vi "HGB2-SpeedControl_Rev00.vi"(11 "Set Speed":dbl format="%#_13g") -> (3 "Speed Control Output":dbl)   [LabVIEW 2016]
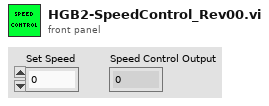
[diagram p1: front panel]
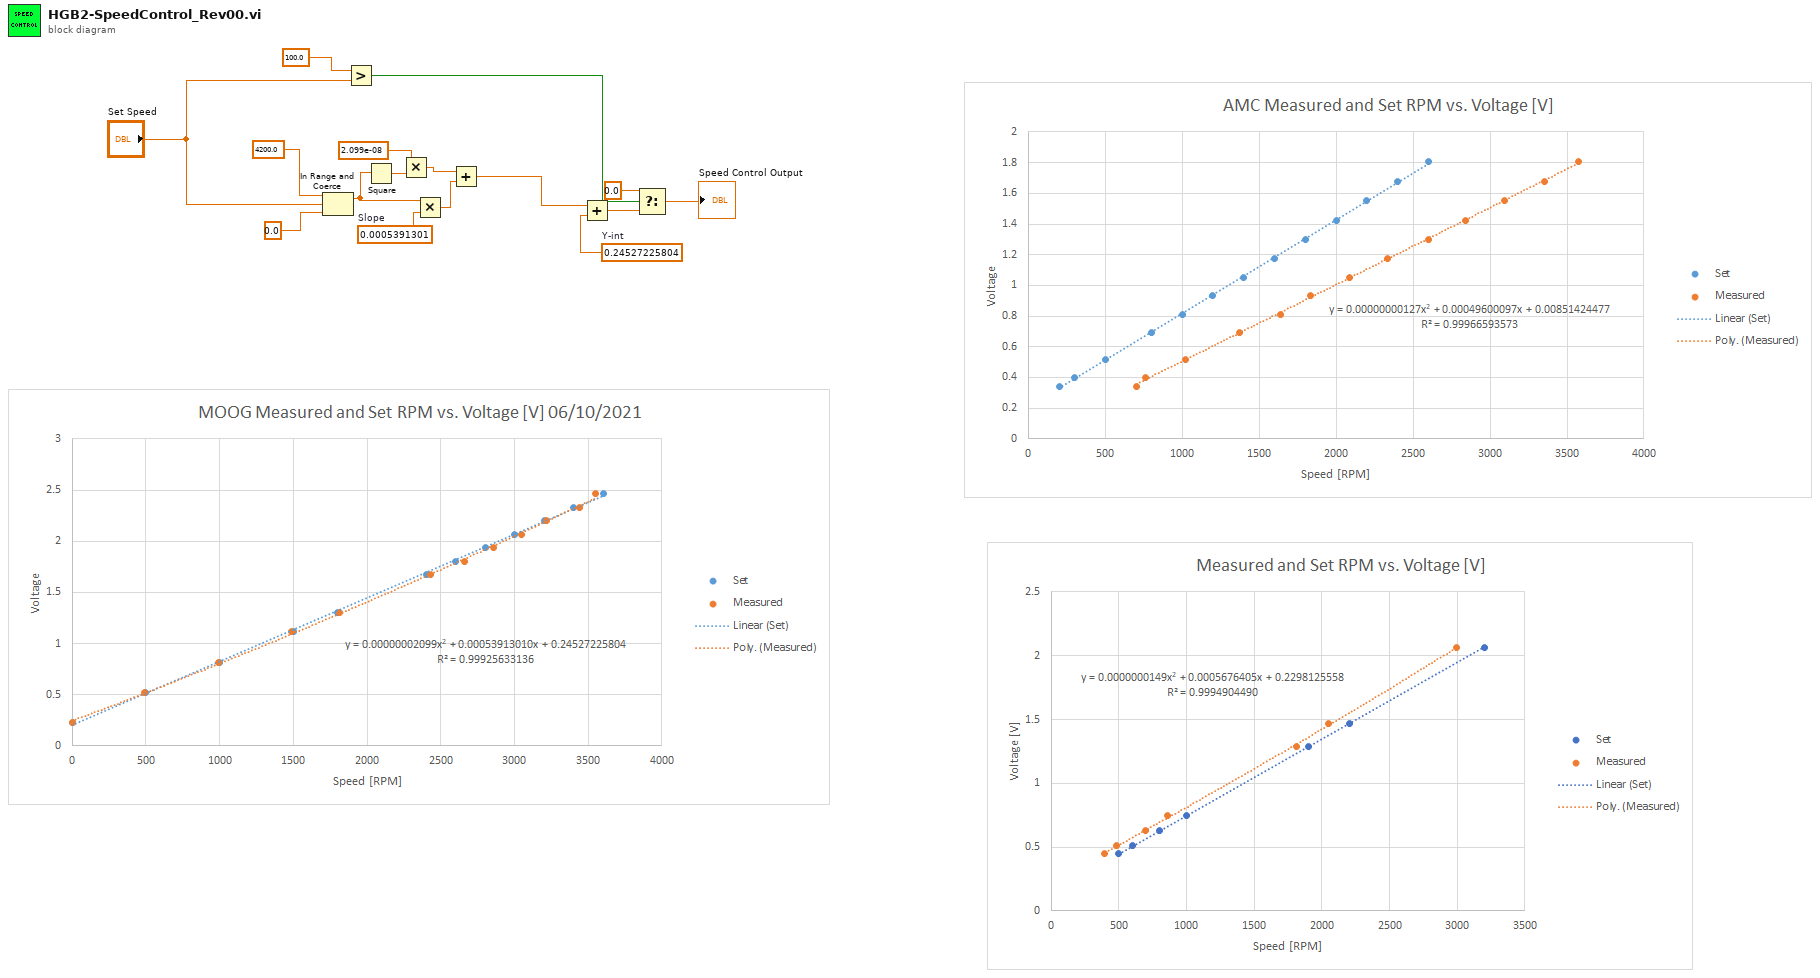
[diagram p0: block diagram]
diagram:
  w8 = 0.24527225804  # Y-int
  w7 = 0.0005391301  # Slope
  n1 = In Range and Coerce(upper limit=4200.0, x="Set Speed", lower limit=0.0) -> (coerced(x)=w6:dbl)  [unwired: 1 out]
  n2 = Greater?(x=100.0, y="Set Speed") -> (0:w15:bool)
  n3 = Square(x=w6) -> (x^2=w3:dbl)
  n4 = Multiply(x=2.099e-08, y=w3) -> (x*y=w2:dbl)
  n5 = Multiply(x=w6, y=w7) -> (x*y=w5:dbl)
  n6 = Add(x=w2, y=w5) -> (x+y=w4:dbl)
  n7 = Add(x=w4, y=w8) -> (x+y=w11:dbl)
  n8 = Select(t=0.0, s=w15, f=w11) -> (s? t:f=→"Speed Control Output":dbl)
